vi "CO calc loffB.vi"(8 "Flow rate":dbl, 10 "Lambda_t":dbl, 11 "O2 Eq Up":dbl) -> (2 "CO MFR 2":dbl)   [LabVIEW 2011]
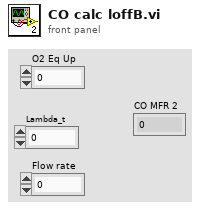
[diagram p1: front panel]
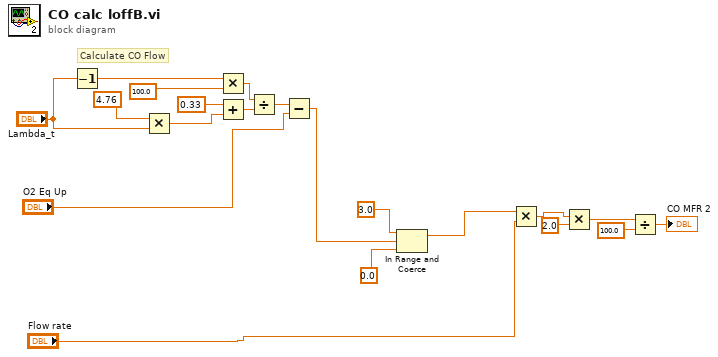
[diagram p0: block diagram]
diagram:
  # "Calculate CO Flow"
  n1 = Decrement(x="Lambda_t") -> (x-1=w20:dbl)
  n2 = Multiply(x=4.76, y="Lambda_t") -> (x*y=w17:dbl)
  n3 = Multiply(x=w20, y=100.0) -> (x*y=w18:dbl)
  n4 = Add(x=0.33, y=w17) -> (x+y=w16:dbl)
  n5 = Divide(x=w18, y=w16) -> (x/y=w7:dbl)
  n6 = Subtract(x=w7, y="O2 Eq Up") -> (x-y=w2:dbl)
  n7 = In Range and Coerce(upper limit=3.0 ("y"), x=w2, lower limit=0.0) -> (coerced(x)=w5:dbl)  [unwired: 1 out]
  n8 = Multiply(x=w5, y="Flow rate") -> (x*y=w8:dbl)
  n9 = Multiply(x=w8, y=2.0) -> (x*y=w14:dbl)
  n10 = Divide(x=w14, y=100.0) -> (x/y=→"CO MFR 2":dbl)
